vi "Drive Process.vi"   [LabVIEW 2013]
uses:
  Drive Global.vi
  <vilib>/Rock Robotics/WPI/Joystick/WPI_JoystickGetSetRefNum.vi
types:
  T1 = typedef "WPI_JoystickDevRef.ctl" = cluster{"Device":T2}
  T2 = typedef "WPI_JoystickDeviceEnum.ctl" = enum16{"USB 1", "USB 2", "USB 3", "USB 4", "Kinect 1", "Kinect 2"}
  T3 = typedef "WPI_JoystickButtonState.ctl" = cluster{"Button 1":bool, "Button 2":bool, "Button 3":bool, "Button 4":bool, "Button 5":bool, "Button 6":bool, "Button 7":bool, "Button 8":bool, "Button 9":bool, "Button 10":bool, "Button 11":bool, "Button 12":bool}
  T4 = cluster{"axis 1 (x)":dbl, "axis 2 (y)":dbl, "axis 3 (throttle)":dbl, "axis 4":dbl, "axis 5":dbl, "axis 6":dbl}
  T5 = cluster{"X Axis":dbl, "Y Axis":dbl, "Slow Drive":bool, "Show Off Spin":bool, "Hands Off":bool, "Right Gear Distance":dbl, "Left Gear Distance ":dbl, "Right Gear RPM":dbl, "Left Gear RPM":dbl}
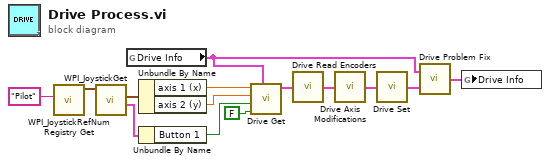
[diagram p0: block diagram]
diagram:
  n1 = call <vilib>:"WPI_JoystickRefNum Registry Get.vi"("refnum name"="Pilot" ("Joystick Name")) -> ("JoystickDevRef"=w8:T1)  [unwired: 9 in, 1 out]
  n2 = call <vilib>:"WPI_JoystickGet.vi"("JoystickDevRef"=w8) -> ("Buttons"=w5:T3, "Axes"=w6:T4)  [unwired: 4 in, 1 out]
  n3 = global read "Drive Global.vi" "Drive Info"() -> (w10:T5)
  n4 = Unbundle By Name(w6) -> ("axis 1 (x)"=w4:dbl, "axis 2 (y)"=w3:dbl)
  n5 = Unbundle By Name(w5) -> ("Button 1"=w2:bool)
  n6 = call "Drive Get.vi"("Drive Info In"=w10, "Show off spin"=FALSE, "Slow Drive"=w2, "Y - Axis"=w3, "X - Axis"=w4) -> ("Drive Info Out"=w9:T5)  [unwired: 6 in]
  n7 = call "Drive Read Encoders.vi"("Drive Info"=w9) -> ("Drive Out"=w11:T5)
  n8 = call "Drive Axis Modifications.vi"("Drive Info In"=w11) -> ("Drive Info Out"=w13:T5)
  n9 = call "Drive Set.vi"("Drive Info In"=w13) -> ("Drive Info Out"=w12:T5)
  n10 = call "Drive Problem Fix.vi"("Drive Info Modified"=w12, "Drive Info Original"=w10) -> ("Drive Info Fixed"=w14:T5)
  n11 = global write "Drive Global.vi" "Drive Info"(w14) -> ()
